vi "Test Set Plugin Parameter.vi"(8 "error in (no error)":errorcluster, 11 "Configuration Manager Test in":refnum<class "Configuration Manager Test.lvclass">) -> (0 "error out":errorcluster, 3 "Configuration Manager Test out":refnum<class "Configuration Manager Test.lvclass">)   [LabVIEW 2020, in "Configuration Manager Test.lvclass"]
uses:
  Configuration Manager Test.lvclass
  Configuration Manager Test.lvclass/Configuration Manager Test.ctl
  source/User Interface/Configuration Manager/Configuration Manager.lvclass
  da4b3e93-04f0-485b-8eef-eaf6a6b0a3f6.vi
  source/Plugins/Plugin/Plugin.lvclass
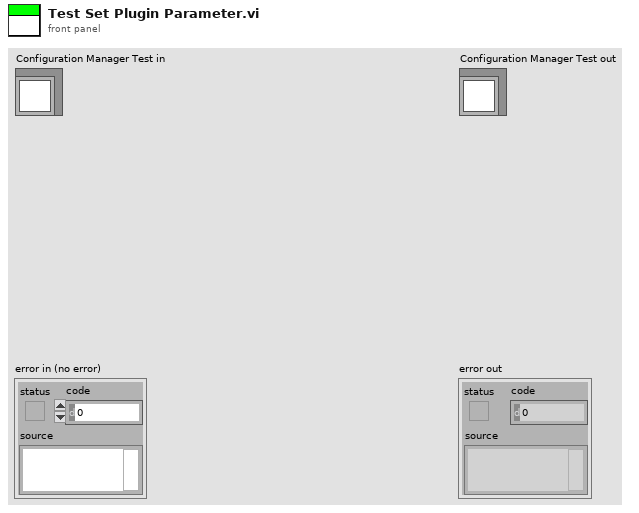
[diagram p1: front panel]
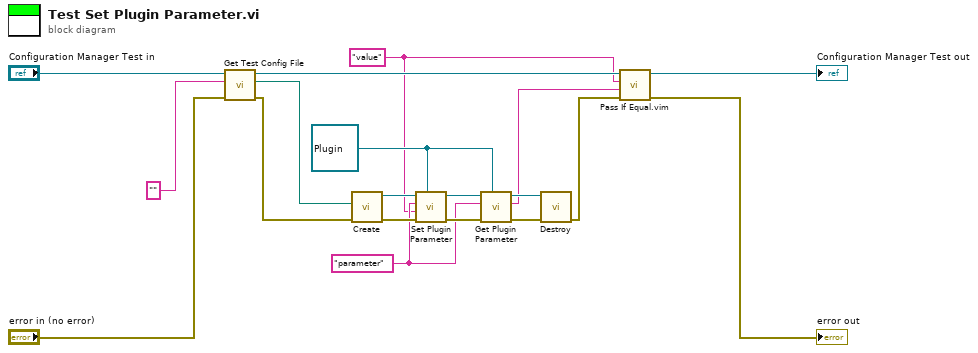
[diagram p0: block diagram]
diagram:
  w2 = "parameter" ("Name")
  w3 = refnum<class "Plugin.lvclass"> refnum ("Plugin.lvclass")
  w1 = "value" ("Report Path")
  n1 = call "Get Test Config File.vi"("error in (no error)"="error in (no error)", "File Content"="", "Configuration Manager Test in"="Configuration Manager Test in") -> ("error out"=w13:errorcluster, "File Path"=w8:path, "Configuration Manager Test out"=w10:refnum<class "Configuration Manager Test.lvclass">)  [unwired: 6 in]
  n2 = call "Create.vi"("error in (no error)"=w13, "configuration file path"=w8) -> ("error out"=w16:errorcluster, "Configuration Manager out"=w5:refnum<class "Configuration Manager.lvclass">)  [unwired: 8 in]
  n3 = call "Set Plugin Parameter.vi"("Plugin.lvclass"=w3, "error in (no error)"=w16, "Value"=w1, "Name"=w2, "Configuration Manager in"=w5) -> ("error out"=w6:errorcluster, "Configuration Manager out"=w4:refnum<class "Configuration Manager.lvclass">)  [unwired: 5 in]
  n4 = call "Get Plugin Parameter.vi"("Plugin.lvclass"=w3, "error in (no error)"=w6, "Name"=w2, "Configuration Manager in"=w4) -> ("error out"=w14:errorcluster, "Value"=w7:string, "Configuration Manager out"=w15:refnum<class "Configuration Manager.lvclass">)  [unwired: 5 in]
  n5 = call "Destroy.vi"("error in (no error)"=w14, "Configuration Manager In"=w15) -> ("error out"=w12:errorcluster)  [unwired: 9 in]
  n6 = call "Pass If Equal.vim"("error in (no error)"=w12, "Actual"=w7, "Expected"=w1, "LUnit Test Case In"=w10) -> ("error out"=→"error out":errorcluster, "LUnit Test Case Out"=→"Configuration Manager Test out":refnum<class "Configuration Manager Test.lvclass">)  [unwired: 6 in]
